vi "Shock&Dyanamics Laboratory - DROPBEAR_June2022_Rev3.vi"() -> ()   [LabVIEW 2019] (continued)
            n8 = property on="Longitudinal Strain Rate" class="WFGraph (strict)"(error in=w28, "Value"=w25) -> (error out=w27:errorcluster)  [unwired: 1 in, 1 out]
            n9 = property on="Velocity" class="WFGraph (strict)"(error in=w27, "Value"=w25) -> (error out=w26:errorcluster)  [unwired: 1 in, 1 out]
            n10 = property on="Acceleration" class="WFGraph (strict)"(error in=w26, "Value"=w25) -> (error out=w24:errorcluster)  [unwired: 1 in, 1 out]
            n11 = property on="Triggered" class="Bool (strict)"(error in=w24, "Value"=w16) -> (error out=w23:errorcluster)  [unwired: 1 in, 1 out]
            n12 = property on="Armed" class="Bool (strict)"(error in=w23, "Value"=w16) -> (error out=w21:errorcluster)  [unwired: 1 in, 1 out]
            n13 = property on="Striker Velocity (m/s)" class="DigNum (strict)"(error in=w21, "Value"=0.0 ("Striker Velocity")) -> (error out=w19:errorcluster)  [unwired: 1 in, 1 out]
            n14 = To Variant(anything=w16) -> (Variant=w17:variant)
            n15 = property on="Load Test Data 2" class="Bool"(error in=w19, "Value"=w17) -> (error out=w18:errorcluster)  [unwired: 1 in, 1 out]
            "Finished Saving Data" <- w16
          }
          frame "Idle" {
            w31 = FALSE ("Finished Saving Data")
            # "Wait for the user to press a button or change a parameter and then act accordingly"
            n16 = property on="Finished Saving Data" class="Bool (strict)"(error in=w34, "Value"=w31) -> (error out=w33:errorcluster)  [unwired: 1 in, 1 out]
            n17 = event shown="[2] \"Trigger (Yes if on)\", \"\": Value Change" {
              selector: _ -> [_ _ _ _ _ _ _ _ _ _ _ _ _ _ _ _ _]
              dyn-events: _ -> [_ _ _ _ _ _ _ _ _ _ _ _ _ _ _ _ _]
              timeout: _ -> [_ _ _ _ _ _ _ _ _ _ _ _ _ _ _ _ _]
              tunnel: [w36 32CHDAQ_-_Cases."Save Data" ("Program State") 32CHDAQ_-_Cases."Idle" ("Program State") 32CHDAQ_-_Cases."Idle" ("Program State") 32CHDAQ_-_Cases."Idle" ("Program State") 32CHDAQ_-_Cases."Idle" ("Program State") 32CHDAQ_-_Cases."Idle" ("Program State") 32CHDAQ_-_Cases."Idle" ("Program State") 32CHDAQ_-_Cases."Load Data" ("Program State") 32CHDAQ_-_Cases."Idle" ("Program State") 32CHDAQ_-_Cases."Idle" ("Program State") 32CHDAQ_-_Cases."Initialize" ("Program State") 32CHDAQ_-_Cases."Initialize" ("Program State") 32CHDAQ_-_Cases."Idle" ("Program State") 32CHDAQ_-_Cases."Execute" ("Program State") 32CHDAQ_-_Cases."Idle" ("Program State") 32CHDAQ_-_Cases."Idle" ("Program State")] -> w35
              event "End Program": Value Change {
                # "Prompt User to Save Data File"
                # "Set the state to End if data is saved"
                n18 = event-data() -> ()  [unwired: 1 in, 5 out]
                n19 = Two Button Dialog(message="Did you save your data?", 1:"No" ("F button name (\"Cancel\")"), 2:"Yes" ("T button name (\"OK\")")) -> (T button?=w37:bool)
                n20 = case shown="False" w37 {
                  tunnel: [w41 32CHDAQ_-_Cases."End" ("Program State")] -> w36
                  frame False {
                    n21 = Two Button Dialog(message="Do you want to save your data?", 1:"No" ("F button name (\"Cancel\")"), 2:"Yes" ("T button name (\"OK\")")) -> (T button?=w42:bool)
                    n22 = case shown="True" w42 {
                      tunnel: [32CHDAQ_-_Cases."End" ("Program State") 32CHDAQ_-_Cases."Save Data" ("Program State")] -> w41
                      frame False {
                      }
                      frame True {
                      }
                    }
                  }
                  frame True {
                  }
                }
              }
              event "Save Data?": Value Change {
                # "Save Button"
                n23 = event-data() -> ()  [unwired: 1 in, 6 out]
              }
              event "Trigger (Yes if on)": Value Change {
                n24 = event-data() -> ()  [unwired: 1 in, 6 out]
                n25 = case shown="\"Trigger Settings\", Default" "?" {
                  tunnel: [w59 w60] -> w52
                  frame "Trigger Settings", Default {
                    w59 = TRUE ("Trigger (Yes if on)")
                    n26 = property on="Trigger (Yes if on)" class="Bool (strict)"("Value"=w59) -> ()  [unwired: 2 in, 2 out]
                  }
                  frame "Continuous" {
                    w60 = FALSE ("Trigger (Yes if on)")
                    n27 = property on="Trigger (Yes if on)" class="Bool (strict)"("Value"=w60) -> ()  [unwired: 2 in, 2 out]
                  }
                }
                n28 = case shown="\"Continuous\"" "?" {
                  tunnel: [T6."Raw Data" ("View Data") T6."Continuous" ("View Data")] -> w50
                  frame "Trigger Settings", Default {
                  }
                  frame "Continuous" {
                  }
                }
                n29 = case shown="True" w52 {
                  tunnel: [T1."Continuous Settings" T1."Trigger Settings"] -> w53
                  frame False {
                  }
                  frame True {
                  }
                }
                "Enum" <- w53
                n30 = property on="View Data" class="TabCtl (strict)"("Value"=w50) -> ()  [unwired: 2 in, 2 out]
              }
              event "Enable Ch 15", "Enable Ch 14", "Enable Ch 13", "Enable Ch 12", "Enable Ch 11", "Enable Ch 10", "Enable Ch 9", "Enable Ch 8", "Enable Ch 7", "Enable Ch 6", "Enable Ch 5", "Enable Ch 4", "Enable Ch 3", "Enable Ch 2", "Enable Ch 1", "Enable Ch 16", "Enable Ch 17", "Enable Ch 18", "Enable Ch 19", "Enable Ch 20", "Enable Ch 21", "Enable Ch 22", "Enable Ch 23", "Enable Ch 24", "Enable Ch 25", "Enable Ch 26", "Enable Ch 27", "Enable Ch 28", "Enable Ch 29", "Enable Ch 30", "Enable Ch 31", "First Pulse", "Separated": Value Change {
                # "Turn Channels on/off and enable/diable assoicated inputs"
                n31 = event-data() -> ()  [unwired: 1 in, 5 out]
                n32 = property on="Enable Ch 17" class="Bool (strict)"() -> ("Value"=w213:bool)  [unwired: 2 in, 2 out]
                "LED Enable Ch 17" <- w213
                n33 = property on="Enable Ch 18" class="Bool (strict)"() -> ("Value"=w212:bool)  [unwired: 2 in, 2 out]
                "LED Enable Ch 18" <- w212
                n34 = property on="Enable Ch 19" class="Bool (strict)"() -> ("Value"=w211:bool)  [unwired: 2 in, 2 out]
                "LED Enable Ch 19" <- w211
                n35 = property on="Enable Ch 16" class="Bool (strict)"() -> ("Value"=w214:bool)  [unwired: 2 in, 2 out]
                "LED Enable Ch 16" <- w214
                n36 = property on="Enable Ch 23" class="Bool (strict)"() -> ("Value"=w207:bool)  [unwired: 2 in, 2 out]
                "LED Enable Ch 23" <- w207
                n37 = property on="Enable Ch 20" class="Bool (strict)"() -> ("Value"=w210:bool)  [unwired: 2 in, 2 out]
                "LED Enable Ch 20" <- w210
                n38 = property on="Enable Ch 21" class="Bool (strict)"() -> ("Value"=w209:bool)  [unwired: 2 in, 2 out]
                "LED Enable Ch 21" <- w209
                n39 = property on="Enable Ch 22" class="Bool (strict)"() -> ("Value"=w208:bool)  [unwired: 2 in, 2 out]
                "LED Enable Ch 22" <- w208
                n40 = property on="Enable Ch 29" class="Bool (strict)"() -> ("Value"=w201:bool)  [unwired: 2 in, 2 out]
                "LED Enable Ch 29" <- w201
                n41 = property on="Enable Ch 28" class="Bool (strict)"() -> ("Value"=w202:bool)  [unwired: 2 in, 2 out]
                "LED Enable Ch 28" <- w202
                n42 = property on="Enable Ch 30" class="Bool (strict)"() -> ("Value"=w200:bool)  [unwired: 2 in, 2 out]
                "LED Enable Ch 30" <- w200
                n43 = property on="Enable Ch 31" class="Bool (strict)"() -> ("Value"=w199:bool)  [unwired: 2 in, 2 out]
                "LED Enable Ch 31" <- w199
                n44 = property on="Enable Ch 15" class="Bool (strict)"() -> ("Value"=w222:bool)  [unwired: 2 in, 2 out]
                "LED Enable Ch 15" <- w222
                n45 = property on="Enable Ch 27" class="Bool (strict)"() -> ("Value"=w203:bool)  [unwired: 2 in, 2 out]
                "LED Enable Ch 27" <- w203
                n46 = property on="Enable Ch 26" class="Bool (strict)"() -> ("Value"=w204:bool)  [unwired: 2 in, 2 out]
                "LED Enable Ch 26" <- w204
                n47 = property on="Enable Ch 24" class="Bool (strict)"() -> ("Value"=w206:bool)  [unwired: 2 in, 2 out]
                "LED Enable Ch 24" <- w206
                n48 = property on="Enable Ch 25" class="Bool (strict)"() -> ("Value"=w205:bool)  [unwired: 2 in, 2 out]
                "LED Enable Ch 25" <- w205
                n49 = property on="Enable Ch 1" class="Bool (strict)"() -> ("Value"=w363:bool)  [unwired: 2 in, 2 out]
                "LED Enable Ch 1" <- w363
                n50 = property on="Enable Ch 2" class="Bool (strict)"() -> ("Value"=w338:bool)  [unwired: 2 in, 2 out]
                "LED Enable Ch 2" <- w338
                n51 = property on="Enable Ch 3" class="Bool (strict)"() -> ("Value"=w337:bool)  [unwired: 2 in, 2 out]
                "LED Enable Ch 3" <- w337
                n52 = property on="Enable Ch 4" class="Bool (strict)"() -> ("Value"=w336:bool)  [unwired: 2 in, 2 out]
                "LED Enable Ch 4" <- w336
                n53 = property on="Enable Ch 5" class="Bool (strict)"() -> ("Value"=w322:bool)  [unwired: 2 in, 2 out]
                "LED Enable Ch 5" <- w322
                n54 = property on="Enable Ch 6" class="Bool (strict)"() -> ("Value"=w303:bool)  [unwired: 2 in, 2 out]
                "LED Enable Ch 6" <- w303
                n55 = property on="Enable Ch 7" class="Bool (strict)"() -> ("Value"=w302:bool)  [unwired: 2 in, 2 out]
                "LED Enable Ch 7" <- w302
                n56 = property on="Enable Ch 8" class="Bool (strict)"() -> ("Value"=w274:bool)  [unwired: 2 in, 2 out]
                "LED Enable Ch 8" <- w274
                n57 = property on="Enable Ch 9" class="Bool (strict)"() -> ("Value"=w273:bool)  [unwired: 2 in, 2 out]
                "LED Enable Ch 9" <- w273
                n58 = property on="Enable Ch 10" class="Bool (strict)"() -> ("Value"=w272:bool)  [unwired: 2 in, 2 out]
                "LED Enable Ch 10" <- w272
                n59 = property on="Enable Ch 11" class="Bool (strict)"() -> ("Value"=w226:bool)  [unwired: 2 in, 2 out]
                "LED Enable Ch 11" <- w226
                n60 = property on="Enable Ch 12" class="Bool (strict)"() -> ("Value"=w225:bool)  [unwired: 2 in, 2 out]
                "LED Enable Ch 12" <- w225
                n61 = property on="Enable Ch 13" class="Bool (strict)"() -> ("Value"=w224:bool)  [unwired: 2 in, 2 out]
                "LED Enable Ch 13" <- w224
                n62 = property on="Enable Ch 14" class="Bool (strict)"() -> ("Value"=w223:bool)  [unwired: 2 in, 2 out]
                "LED Enable Ch 14" <- w223
                n63 = Bundle("Enable Ch 1"=TRUE, "Value"=w363, "Value"=w338, "Value"=w337, "Value"=w336, "Value"=w322, "Value"=w303, "Value"=w302, "Value"=w274, "Value"=w273, "Value"=w272, "Value"=w226, "Value"=w225, "Value"=w224, "Value"=w223, "Value"=w222, "Value"=w214, "Value"=w213, "Value"=w212, "Value"=w211, "Value"=w210, "Value"=w209, "Value"=w208, "Value"=w207, "Value"=w206, "Value"=w205, "Value"=w204, "Value"=w203, "Value"=w202, "Value"=w201, "Value"=w200, "Value"=w199) -> ()  [unwired: 1 in, 1 out]
                n64 = case shown="False" w212 {
                  tunnel: [w661 T42."Enabled" ("Disabled")] -> w178
                  tunnel: [w662 w665] -> w186
                  frame False {
                    w661 = T42."Disabled and Grayed Out" ("Disabled")
                    n65 = property on="SG Pair 18" class="Bool (strict)"("DisabledEnum"=w661) -> (error out=w660:errorcluster)  [unwired: 2 in, 1 out]
                    n66 = property on="SG Pair Ch 18" class="Enum (strict)"(error in=w660, "DisabledEnum"=w661) -> (error out=w659:errorcluster)  [unwired: 1 in, 1 out]
                    n67 = property on="PF Chassis 18" class="DigNum (strict)"(error in=w659, "DisabledEnum"=w661) -> (error out=w664:errorcluster)  [unwired: 1 in, 1 out]
                    n68 = property on="PF Card 18" class="DigNum (strict)"(error in=w664, "DisabledEnum"=w661) -> (error out=w663:errorcluster)  [unwired: 1 in, 1 out]
                    n69 = property on="PF Channel 18" class="DigNum (strict)"(error in=w663, "DisabledEnum"=w661) -> (error out=w662:errorcluster)  [unwired: 1 in, 1 out]
                  }
                  frame True {
                    n70 = stacked-sequence {
                      tunnel: [w669 _] -> w665
                      frame #0 {
                        n71 = property on="PF Condition 18" class="Bool (strict)"() -> (error out=w668:errorcluster, "Value"=w667:bool)  [unwired: 2 in, 1 out]
                        n72 = case shown="True" w667 {
                          tunnel: [T42."Disabled and Grayed Out" ("Disabled") T42."Enabled" ("Disabled")] -> w672
                          frame False {
                          }
                          frame True {
                          }
                        }
                        n73 = property on="PF Chassis 18" class="DigNum (strict)"(error in=w668, "DisabledEnum"=w672) -> (error out=w671:errorcluster)  [unwired: 1 in, 1 out]
                        n74 = property on="PF Card 18" class="DigNum (strict)"(error in=w671, "DisabledEnum"=w672) -> (error out=w670:errorcluster)  [unwired: 1 in, 1 out]
                        n75 = property on="PF Channel 18" class="DigNum (strict)"(error in=w670, "DisabledEnum"=w672) -> (error out=w669:errorcluster)  [unwired: 1 in, 1 out]
                      }
                      frame #1 {
                        n76 = property on="Signal Type 18" class="Enum (strict)"() -> (error out=w677:errorcluster, "Value"=w678:T8)  [unwired: 2 in, 1 out]
                        n77 = case shown="\"Voltage\", Default" w678 {
                          tunnel: [T42."Enabled" ("Disabled") T42."Disabled and Grayed Out" ("Disabled")] -> w676
                          frame "Strain" {
                          }
                          frame "Voltage", Default {
                          }
                        }
                        n78 = property on="SG Pair 18" class="Bool (strict)"(error in=w677, "DisabledEnum"=w676) -> (error out=w675:errorcluster)  [unwired: 1 in, 1 out]
                        n79 = property on="SG Pair Ch 18" class="Enum (strict)"(error in=w675, "DisabledEnum"=w676) -> ()  [unwired: 1 in, 2 out]
                      }
                    }
                  }
                }
                n80 = case shown="False" w211 {
                  tunnel: [w639 T42."Enabled" ("Disabled")] -> w177
                  tunnel: [w642 w643] -> w169
                  frame False {
                    w639 = T42."Disabled and Grayed Out" ("Disabled")
                    n81 = property on="SG Pair 19" class="Bool (strict)"("DisabledEnum"=w639) -> (error out=w638:errorcluster)  [unwired: 2 in, 1 out]
                    n82 = property on="SG Pair Ch 19" class="Enum (strict)"(error in=w638, "DisabledEnum"=w639) -> (error out=w637:errorcluster)  [unwired: 1 in, 1 out]
                    n83 = property on="PF Chassis 19" class="DigNum (strict)"(error in=w637, "DisabledEnum"=w639) -> (error out=w640:errorcluster)  [unwired: 1 in, 1 out]
                    n84 = property on="PF Card 19" class="DigNum (strict)"(error in=w640, "DisabledEnum"=w639) -> (error out=w641:errorcluster)  [unwired: 1 in, 1 out]
                    n85 = property on="PF Channel 19" class="DigNum (strict)"(error in=w641, "DisabledEnum"=w639) -> (error out=w642:errorcluster)  [unwired: 1 in, 1 out]
                  }
                  frame True {
                    n86 = stacked-sequence {
                      tunnel: [w648 _] -> w643
                      frame #0 {
                        n87 = property on="PF Condition 19" class="Bool (strict)"() -> (error out=w645:errorcluster, "Value"=w650:bool)  [unwired: 2 in, 1 out]
                        n88 = case shown="True" w650 {
                          tunnel: [T42."Disabled and Grayed Out" ("Disabled") T42."Enabled" ("Disabled")] -> w649
                          frame False {
                          }
                          frame True {
                          }
                        }
                        n89 = property on="PF Chassis 19" class="DigNum (strict)"(error in=w645, "DisabledEnum"=w649) -> (error out=w646:errorcluster)  [unwired: 1 in, 1 out]
                        n90 = property on="PF Card 19" class="DigNum (strict)"(error in=w646, "DisabledEnum"=w649) -> (error out=w647:errorcluster)  [unwired: 1 in, 1 out]
                        n91 = property on="PF Channel 19" class="DigNum (strict)"(error in=w647, "DisabledEnum"=w649) -> (error out=w648:errorcluster)  [unwired: 1 in, 1 out]
                      }
                      frame #1 {
                        n92 = property on="Signal Type 19" class="Enum (strict)"() -> (error out=w656:errorcluster, "Value"=w655:T8)  [unwired: 2 in, 1 out]
                        n93 = case shown="\"Voltage\", Default" w655 {
                          tunnel: [T42."Enabled" ("Disabled") T42."Disabled and Grayed Out" ("Disabled")] -> w654
                          frame "Strain" {
                          }
                          frame "Voltage", Default {
                          }
                        }
                        n94 = property on="SG Pair 19" class="Bool (strict)"(error in=w656, "DisabledEnum"=w654) -> (error out=w653:errorcluster)  [unwired: 1 in, 1 out]
                        n95 = property on="SG Pair Ch 19" class="Enum (strict)"(error in=w653, "DisabledEnum"=w654) -> ()  [unwired: 1 in, 2 out]
                      }
                    }
                  }
                }
                n96 = case shown="True" w363 {
                  tunnel: [w1035 T42."Enabled" ("Disabled")] -> w365
                  tunnel: [w1036 w1039] -> w335
                  frame False {
                    w1035 = T42."Disabled and Grayed Out" ("Disabled")
                    n97 = property on="SG Pair 1" class="Bool (strict)"("DisabledEnum"=w1035) -> (error out=w1034:errorcluster)  [unwired: 2 in, 1 out]
                    n98 = property on="SG Pair Ch 1" class="Enum (strict)"(error in=w1034, "DisabledEnum"=w1035) -> (error out=w1033:errorcluster)  [unwired: 1 in, 1 out]
                    n99 = property on="PF Chassis 1" class="DigNum (strict)"(error in=w1033, "DisabledEnum"=w1035) -> (error out=w1038:errorcluster)  [unwired: 1 in, 1 out]
                    n100 = property on="PF Card 1" class="DigNum (strict)"(error in=w1038, "DisabledEnum"=w1035) -> (error out=w1037:errorcluster)  [unwired: 1 in, 1 out]
                    n101 = property on="PF Channel 1" class="DigNum (strict)"(error in=w1037, "DisabledEnum"=w1035) -> (error out=w1036:errorcluster)  [unwired: 1 in, 1 out]
                  }
                  frame True {
                    n102 = stacked-sequence {
                      tunnel: [w1041 _] -> w1039
                      frame #0 {
                        n103 = property on="PF Condition 1" class="Bool (strict)"() -> (error out=w1046:errorcluster, "Value"=w1043:bool)  [unwired: 2 in, 1 out]
                        n104 = case shown="True" w1043 {
                          tunnel: [T42."Disabled and Grayed Out" ("Disabled") T42."Enabled" ("Disabled")] -> w1042
                          frame False {
                          }
                          frame True {
                          }
                        }
                        n105 = property on="PF Chassis 1" class="DigNum (strict)"(error in=w1046, "DisabledEnum"=w1042) -> (error out=w1045:errorcluster)  [unwired: 1 in, 1 out]
                        n106 = property on="PF Card 1" class="DigNum (strict)"(error in=w1045, "DisabledEnum"=w1042) -> (error out=w1044:errorcluster)  [unwired: 1 in, 1 out]
                        n107 = property on="PF Channel 1" class="DigNum (strict)"(error in=w1044, "DisabledEnum"=w1042) -> (error out=w1041:errorcluster)  [unwired: 1 in, 1 out]
                      }
                      frame #1 {
                        n108 = property on="Signal Type 1" class="Enum (strict)"() -> (error out=w1052:errorcluster, "Value"=w1051:T8)  [unwired: 2 in, 1 out]
                        n109 = case shown="\"Strain\"" w1051 {
                          tunnel: [T42."Enabled" ("Disabled") T42."Disabled and Grayed Out" ("Disabled")] -> w1050
                          frame "Strain" {
                          }
                          frame "Voltage", Default {
                          }
                        }
                        n110 = property on="SG Pair 1" class="Bool (strict)"(error in=w1052, "DisabledEnum"=w1050) -> (error out=w1049:errorcluster)  [unwired: 1 in, 1 out]
                        n111 = property on="SG Pair Ch 1" class="Enum (strict)"(error in=w1049, "DisabledEnum"=w1050) -> ()  [unwired: 1 in, 2 out]
                      }
                    }
                  }
                }
                n112 = case shown="False" w338 {
                  tunnel: [w1011 T42."Enabled" ("Disabled")] -> w356
                  tunnel: [w1014 w1017] -> w334
                  frame False {
                    w1011 = T42."Disabled and Grayed Out" ("Disabled")
                    n113 = property on="SG Pair 2" class="Bool (strict)"("DisabledEnum"=w1011) -> (error out=w1013:errorcluster)  [unwired: 2 in, 1 out]
                    n114 = property on="SG Pair Ch 2" class="Enum (strict)"(error in=w1013, "DisabledEnum"=w1011) -> (error out=w1012:errorcluster)  [unwired: 1 in, 1 out]
                    n115 = property on="PF Chassis 2" class="DigNum (strict)"(error in=w1012, "DisabledEnum"=w1011) -> (error out=w1016:errorcluster)  [unwired: 1 in, 1 out]
                    n116 = property on="PF Card 2" class="DigNum (strict)"(error in=w1016, "DisabledEnum"=w1011) -> (error out=w1015:errorcluster)  [unwired: 1 in, 1 out]
                    n117 = property on="PF Channel 2" class="DigNum (strict)"(error in=w1015, "DisabledEnum"=w1011) -> (error out=w1014:errorcluster)  [unwired: 1 in, 1 out]
                  }
                  frame True {
                    n118 = stacked-sequence {
                      tunnel: [w1019 _] -> w1017
                      frame #0 {
                        n119 = property on="PF Condition 2" class="Bool (strict)"() -> (error out=w1020:errorcluster, "Value"=w1023:bool)  [unwired: 2 in, 1 out]
                        n120 = case shown="True" w1023 {
                          tunnel: [T42."Disabled and Grayed Out" ("Disabled") T42."Enabled" ("Disabled")] -> w1024
                          frame False {
                          }
                          frame True {
                          }
                        }
                        n121 = property on="PF Chassis 2" class="DigNum (strict)"(error in=w1020, "DisabledEnum"=w1024) -> (error out=w1021:errorcluster)  [unwired: 1 in, 1 out]
                        n122 = property on="PF Card 2" class="DigNum (strict)"(error in=w1021, "DisabledEnum"=w1024) -> (error out=w1022:errorcluster)  [unwired: 1 in, 1 out]
                        n123 = property on="PF Channel 2" class="DigNum (strict)"(error in=w1022, "DisabledEnum"=w1024) -> (error out=w1019:errorcluster)  [unwired: 1 in, 1 out]
                      }
                      frame #1 {
                        n124 = property on="Signal Type 2" class="Enum (strict)"() -> (error out=w1030:errorcluster, "Value"=w1029:T8)  [unwired: 2 in, 1 out]
                        n125 = case shown="\"Voltage\", Default" w1029 {
                          tunnel: [T42."Enabled" ("Disabled") T42."Disabled and Grayed Out" ("Disabled")] -> w1028
                          frame "Strain" {
                          }
                          frame "Voltage", Default {
                          }
                        }
                        n126 = property on="SG Pair 2" class="Bool (strict)"(error in=w1030, "DisabledEnum"=w1028) -> (error out=w1027:errorcluster)  [unwired: 1 in, 1 out]
                        n127 = property on="SG Pair Ch 2" class="Enum (strict)"(error in=w1027, "DisabledEnum"=w1028) -> ()  [unwired: 1 in, 2 out]
                      }
                    }
                  }
                }
                n128 = case shown="False" w337 {
                  tunnel: [w991 T42."Enabled" ("Disabled")] -> w348
                  tunnel: [w992 w995] -> w333
                  frame False {
                    w991 = T42."Disabled and Grayed Out" ("Disabled")
                    n129 = property on="SG Pair 3" class="Bool (strict)"("DisabledEnum"=w991) -> (error out=w990:errorcluster)  [unwired: 2 in, 1 out]
                    n130 = property on="SG Pair Ch 3" class="Enum (strict)"(error in=w990, "DisabledEnum"=w991) -> (error out=w989:errorcluster)  [unwired: 1 in, 1 out]
                    n131 = property on="PF Chassis 3" class="DigNum (strict)"(error in=w989, "DisabledEnum"=w991) -> (error out=w994:errorcluster)  [unwired: 1 in, 1 out]
                    n132 = property on="PF Card 3" class="DigNum (strict)"(error in=w994, "DisabledEnum"=w991) -> (error out=w993:errorcluster)  [unwired: 1 in, 1 out]
                    n133 = property on="PF Channel 3" class="DigNum (strict)"(error in=w993, "DisabledEnum"=w991) -> (error out=w992:errorcluster)  [unwired: 1 in, 1 out]
                  }
                  frame True {
                    n134 = stacked-sequence {
                      tunnel: [w997 _] -> w995
                      frame #0 {
                        n135 = property on="PF Condition 3" class="Bool (strict)"() -> (error out=w998:errorcluster, "Value"=w1001:bool)  [unwired: 2 in, 1 out]
                        n136 = case shown="True" w1001 {
                          tunnel: [T42."Disabled and Grayed Out" ("Disabled") T42."Enabled" ("Disabled")] -> w1002
                          frame False {
                          }
                          frame True {
                          }
                        }
                        n137 = property on="PF Chassis 3" class="DigNum (strict)"(error in=w998, "DisabledEnum"=w1002) -> (error out=w999:errorcluster)  [unwired: 1 in, 1 out]
                        n138 = property on="PF Card 3" class="DigNum (strict)"(error in=w999, "DisabledEnum"=w1002) -> (error out=w1000:errorcluster)  [unwired: 1 in, 1 out]
                        n139 = property on="PF Channel 3" class="DigNum (strict)"(error in=w1000, "DisabledEnum"=w1002) -> (error out=w997:errorcluster)  [unwired: 1 in, 1 out]
                      }
                      frame #1 {
                        n140 = property on="Signal Type 3" class="Enum (strict)"() -> (error out=w1008:errorcluster, "Value"=w1007:T8)  [unwired: 2 in, 1 out]
                        n141 = case shown="\"Voltage\", Default" w1007 {
                          tunnel: [T42."Enabled" ("Disabled") T42."Disabled and Grayed Out" ("Disabled")] -> w1006
                          frame "Strain" {
                          }
                          frame "Voltage", Default {
                          }
                        }
                        n142 = property on="SG Pair 3" class="Bool (strict)"(error in=w1008, "DisabledEnum"=w1006) -> (error out=w1005:errorcluster)  [unwired: 1 in, 1 out]
                        n143 = property on="SG Pair Ch 3" class="Enum (strict)"(error in=w1005, "DisabledEnum"=w1006) -> ()  [unwired: 1 in, 2 out]
                      }
                    }
                  }
                }
                n144 = case shown="True" w336 {
                  tunnel: [w969 T42."Enabled" ("Disabled")] -> w340
                  tunnel: [w970 w973] -> w332
                  frame False {
                    w969 = T42."Disabled and Grayed Out" ("Disabled")
                    n145 = property on="SG Pair 4" class="Bool (strict)"("DisabledEnum"=w969) -> (error out=w968:errorcluster)  [unwired: 2 in, 1 out]
                    n146 = property on="SG Pair Ch 4" class="Enum (strict)"(error in=w968, "DisabledEnum"=w969) -> (error out=w967:errorcluster)  [unwired: 1 in, 1 out]
                    n147 = property on="PF Chassis 4" class="DigNum (strict)"(error in=w967, "DisabledEnum"=w969) -> (error out=w972:errorcluster)  [unwired: 1 in, 1 out]
                    n148 = property on="PF Card 4" class="DigNum (strict)"(error in=w972, "DisabledEnum"=w969) -> (error out=w971:errorcluster)  [unwired: 1 in, 1 out]
                    n149 = property on="PF Channel 4" class="DigNum (strict)"(error in=w971, "DisabledEnum"=w969) -> (error out=w970:errorcluster)  [unwired: 1 in, 1 out]
                  }
                  frame True {
                    n150 = stacked-sequence {
                      tunnel: [w975 _] -> w973
                      frame #0 {
                        n151 = property on="PF Condition 4" class="Bool (strict)"() -> (error out=w976:errorcluster, "Value"=w979:bool)  [unwired: 2 in, 1 out]
                        n152 = case shown="True" w979 {
                          tunnel: [T42."Disabled and Grayed Out" ("Disabled") T42."Enabled" ("Disabled")] -> w980
                          frame False {
                          }
                          frame True {
                          }
                        }
                        n153 = property on="PF Chassis 4" class="DigNum (strict)"(error in=w976, "DisabledEnum"=w980) -> (error out=w977:errorcluster)  [unwired: 1 in, 1 out]
                        n154 = property on="PF Card 4" class="DigNum (strict)"(error in=w977, "DisabledEnum"=w980) -> (error out=w978:errorcluster)  [unwired: 1 in, 1 out]
                        n155 = property on="PF Channel 4" class="DigNum (strict)"(error in=w978, "DisabledEnum"=w980) -> (error out=w975:errorcluster)  [unwired: 1 in, 1 out]
                      }
                      frame #1 {
                        n156 = property on="Signal Type 4" class="Enum (strict)"() -> (error out=w986:errorcluster, "Value"=w985:T8)  [unwired: 2 in, 1 out]
                        n157 = case shown="\"Strain\"" w985 {
                          tunnel: [T42."Enabled" ("Disabled") T42."Disabled and Grayed Out" ("Disabled")] -> w984
                          frame "Strain" {
                          }
                          frame "Voltage", Default {
                          }
                        }
                        n158 = property on="SG Pair 4" class="Bool (strict)"(error in=w986, "DisabledEnum"=w984) -> (error out=w983:errorcluster)  [unwired: 1 in, 1 out]
                        n159 = property on="SG Pair Ch 4" class="Enum (strict)"(error in=w983, "DisabledEnum"=w984) -> ()  [unwired: 1 in, 2 out]
                      }
                    }
                  }
                }
                n160 = case shown="True" w322 {
                  tunnel: [w947 T42."Enabled" ("Disabled")] -> w325
                  tunnel: [w948 w951] -> w323
                  frame False {
                    w947 = T42."Disabled and Grayed Out" ("Disabled")
                    n161 = property on="SG Pair 5" class="Bool (strict)"("DisabledEnum"=w947) -> (error out=w946:errorcluster)  [unwired: 2 in, 1 out]
                    n162 = property on="SG Pair Ch 5" class="Enum (strict)"(error in=w946, "DisabledEnum"=w947) -> (error out=w945:errorcluster)  [unwired: 1 in, 1 out]
                    n163 = property on="PF Chassis 5" class="DigNum (strict)"(error in=w945, "DisabledEnum"=w947) -> (error out=w950:errorcluster)  [unwired: 1 in, 1 out]
                    n164 = property on="PF Card 5" class="DigNum (strict)"(error in=w950, "DisabledEnum"=w947) -> (error out=w949:errorcluster)  [unwired: 1 in, 1 out]
                    n165 = property on="PF Channel 5" class="DigNum (strict)"(error in=w949, "DisabledEnum"=w947) -> (error out=w948:errorcluster)  [unwired: 1 in, 1 out]
                  }
                  frame True {
                    n166 = stacked-sequence {
                      tunnel: [w953 _] -> w951
                      frame #0 {
                        n167 = property on="PF Condition 5" class="Bool (strict)"() -> (error out=w954:errorcluster, "Value"=w957:bool)  [unwired: 2 in, 1 out]
                        n168 = case shown="True" w957 {
                          tunnel: [T42."Disabled and Grayed Out" ("Disabled") T42."Enabled" ("Disabled")] -> w958
                          frame False {
                          }
                          frame True {
                          }
                        }
                        n169 = property on="PF Chassis 5" class="DigNum (strict)"(error in=w954, "DisabledEnum"=w958) -> (error out=w955:errorcluster)  [unwired: 1 in, 1 out]
                        n170 = property on="PF Card 4" class="DigNum (strict)"(error in=w955, "DisabledEnum"=w958) -> (error out=w956:errorcluster)  [unwired: 1 in, 1 out]
                        n171 = property on="PF Channel 5" class="DigNum (strict)"(error in=w956, "DisabledEnum"=w958) -> (error out=w953:errorcluster)  [unwired: 1 in, 1 out]
                      }
                      frame #1 {
                        n172 = property on="Signal Type 5" class="Enum (strict)"() -> (error out=w964:errorcluster, "Value"=w963:T8)  [unwired: 2 in, 1 out]
                        n173 = case shown="\"Voltage\", Default" w963 {
                          tunnel: [T42."Enabled" ("Disabled") T42."Disabled and Grayed Out" ("Disabled")] -> w962
                          frame "Strain" {
                          }
                          frame "Voltage", Default {
                          }
                        }
                        n174 = property on="SG Pair 5" class="Bool (strict)"(error in=w964, "DisabledEnum"=w962) -> (error out=w961:errorcluster)  [unwired: 1 in, 1 out]
                        n175 = property on="SG Pair Ch 5" class="Enum (strict)"(error in=w961, "DisabledEnum"=w962) -> ()  [unwired: 1 in, 2 out]
                      }
                    }
                  }
                }
                n176 = case shown="False" w303 {
                  tunnel: [w925 T42."Enabled" ("Disabled")] -> w315
                  tunnel: [w926 w929] -> w313
                  frame False {
                    w925 = T42."Disabled and Grayed Out" ("Disabled")
                    n177 = property on="SG Pair 6" class="Bool (strict)"("DisabledEnum"=w925) -> (error out=w924:errorcluster)  [unwired: 2 in, 1 out]
                    n178 = property on="SG Pair Ch 6" class="Enum (strict)"(error in=w924, "DisabledEnum"=w925) -> (error out=w923:errorcluster)  [unwired: 1 in, 1 out]
                    n179 = property on="PF Chassis 6" class="DigNum (strict)"(error in=w923, "DisabledEnum"=w925) -> (error out=w928:errorcluster)  [unwired: 1 in, 1 out]
                    n180 = property on="PF Card 6" class="DigNum (strict)"(error in=w928, "DisabledEnum"=w925) -> (error out=w927:errorcluster)  [unwired: 1 in, 1 out]
                    n181 = property on="PF Channel 6" class="DigNum (strict)"(error in=w927, "DisabledEnum"=w925) -> (error out=w926:errorcluster)  [unwired: 1 in, 1 out]
                  }
                  frame True {
                    n182 = stacked-sequence {
                      tunnel: [w931 _] -> w929
                      frame #0 {
                        n183 = property on="PF Condition 6" class="Bool (strict)"() -> (error out=w932:errorcluster, "Value"=w935:bool)  [unwired: 2 in, 1 out]
                        n184 = case shown="True" w935 {
                          tunnel: [T42."Disabled and Grayed Out" ("Disabled") T42."Enabled" ("Disabled")] -> w936
                          frame False {
                          }
                          frame True {
                          }
                        }
                        n185 = property on="PF Chassis 6" class="DigNum (strict)"(error in=w932, "DisabledEnum"=w936) -> (error out=w933:errorcluster)  [unwired: 1 in, 1 out]
                        n186 = property on="PF Card 6" class="DigNum (strict)"(error in=w933, "DisabledEnum"=w936) -> (error out=w934:errorcluster)  [unwired: 1 in, 1 out]
                        n187 = property on="PF Channel 6" class="DigNum (strict)"(error in=w934, "DisabledEnum"=w936) -> (error out=w931:errorcluster)  [unwired: 1 in, 1 out]
                      }
                      frame #1 {
                        n188 = property on="Signal Type 6" class="Enum (strict)"() -> (error out=w942:errorcluster, "Value"=w941:T8)  [unwired: 2 in, 1 out]
                        n189 = case shown="\"Voltage\", Default" w941 {
                          tunnel: [T42."Enabled" ("Disabled") T42."Disabled and Grayed Out" ("Disabled")] -> w940
                          frame "Strain" {
                          }
                          frame "Voltage", Default {
                          }
                        }
                        n190 = property on="SG Pair 6" class="Bool (strict)"(error in=w942, "DisabledEnum"=w940) -> (error out=w939:errorcluster)  [unwired: 1 in, 1 out]
                        n191 = property on="SG Pair Ch 6" class="Enum (strict)"(error in=w939, "DisabledEnum"=w940) -> ()  [unwired: 1 in, 2 out]
                      }
                    }
                  }
                }
                n192 = case shown="False" w225 {
                  tunnel: [w793 T42."Enabled" ("Disabled")] -> w256
                  tunnel: [w794 w797] -> w254
                  frame False {
                    w793 = T42."Disabled and Grayed Out" ("Disabled")
                    n193 = property on="SG Pair 12" class="Bool (strict)"("DisabledEnum"=w793) -> (error out=w792:errorcluster)  [unwired: 2 in, 1 out]
                    n194 = property on="SG Pair Ch 12" class="Enum (strict)"(error in=w792, "DisabledEnum"=w793) -> (error out=w791:errorcluster)  [unwired: 1 in, 1 out]
                    n195 = property on="PF Chassis 12" class="DigNum (strict)"(error in=w791, "DisabledEnum"=w793) -> (error out=w796:errorcluster)  [unwired: 1 in, 1 out]
                    n196 = property on="PF Card 12" class="DigNum (strict)"(error in=w796, "DisabledEnum"=w793) -> (error out=w795:errorcluster)  [unwired: 1 in, 1 out]
                    n197 = property on="PF Channel 12" class="DigNum (strict)"(error in=w795, "DisabledEnum"=w793) -> (error out=w794:errorcluster)  [unwired: 1 in, 1 out]
                  }
                  frame True {
                    n198 = stacked-sequence {
                      tunnel: [w799 _] -> w797
                      frame #0 {
                        n199 = property on="PF Condition 12" class="Bool (strict)"() -> (error out=w800:errorcluster, "Value"=w803:bool)  [unwired: 2 in, 1 out]
                        n200 = case shown="True" w803 {
                          tunnel: [T42."Disabled and Grayed Out" ("Disabled") T42."Enabled" ("Disabled")] -> w804
                          frame False {
                          }
                          frame True {
                          }
                        }
                        n201 = property on="PF Chassis 12" class="DigNum (strict)"(error in=w800, "DisabledEnum"=w804) -> (error out=w801:errorcluster)  [unwired: 1 in, 1 out]
                        n202 = property on="PF Card 12" class="DigNum (strict)"(error in=w801, "DisabledEnum"=w804) -> (error out=w802:errorcluster)  [unwired: 1 in, 1 out]
                        n203 = property on="PF Channel 12" class="DigNum (strict)"(error in=w802, "DisabledEnum"=w804) -> (error out=w799:errorcluster)  [unwired: 1 in, 1 out]
                      }
                      frame #1 {
                        n204 = property on="Signal Type 12" class="Enum (strict)"() -> (error out=w810:errorcluster, "Value"=w809:T8)  [unwired: 2 in, 1 out]
                        n205 = case shown="\"Voltage\", Default" w809 {
                          tunnel: [T42."Enabled" ("Disabled") T42."Disabled and Grayed Out" ("Disabled")] -> w808
                          frame "Strain" {
                          }
                          frame "Voltage", Default {
                          }
                        }
                        n206 = property on="SG Pair 12" class="Bool (strict)"(error in=w810, "DisabledEnum"=w808) -> (error out=w807:errorcluster)  [unwired: 1 in, 1 out]
                        n207 = property on="SG Pair Ch 12" class="Enum (strict)"(error in=w807, "DisabledEnum"=w808) -> ()  [unwired: 1 in, 2 out]
                      }
                    }
                  }
                }
                n208 = case shown="False" w224 {
                  tunnel: [w771 T42."Enabled" ("Disabled")] -> w247
                  tunnel: [w772 w775] -> w245
                  frame False {
                    w771 = T42."Disabled and Grayed Out" ("Disabled")
                    n209 = property on="SG Pair 13" class="Bool (strict)"("DisabledEnum"=w771) -> (error out=w770:errorcluster)  [unwired: 2 in, 1 out]
                    n210 = property on="SG Pair Ch 13" class="Enum (strict)"(error in=w770, "DisabledEnum"=w771) -> (error out=w769:errorcluster)  [unwired: 1 in, 1 out]
                    n211 = property on="PF Chassis 13" class="DigNum (strict)"(error in=w769, "DisabledEnum"=w771) -> (error out=w774:errorcluster)  [unwired: 1 in, 1 out]
                    n212 = property on="PF Card 13" class="DigNum (strict)"(error in=w774, "DisabledEnum"=w771) -> (error out=w773:errorcluster)  [unwired: 1 in, 1 out]
                    n213 = property on="PF Channel 13" class="DigNum (strict)"(error in=w773, "DisabledEnum"=w771) -> (error out=w772:errorcluster)  [unwired: 1 in, 1 out]
                  }
                  frame True {
                    n214 = stacked-sequence {
